vi "TEST - Get Array Element TD.vi"(8 "error in (no error)":errorcluster) -> (0 "error out":errorcluster, 2 "pass":bool)   [LabVIEW 2020, in "test_openg_variant.lvlib"]
uses:
  test_openg_variant.lvlib
  source/library/Type Descriptor.ctl
  <vilib>/addons/_JKI Toolkits/Caraya/classes/Assert/Assert True.vi
  source/library/openg_variant.lvlib
  <vilib>/addons/_JKI Toolkits/Caraya/classes/Test/Test.lvclass
  <vilib>/addons/_JKI Toolkits/Caraya/classes/Assert/Assert.lvclass
panel:
  out "Failures":T2(array[cluster])
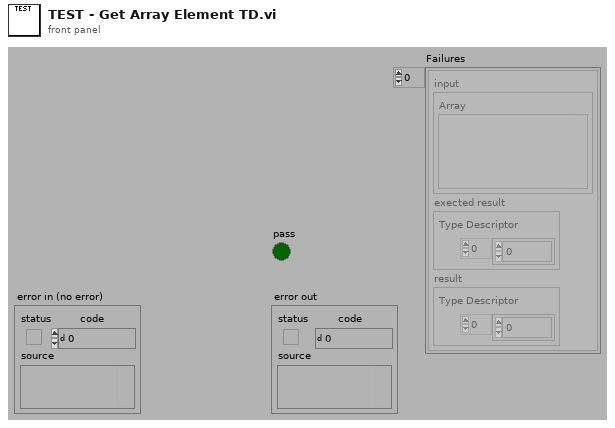
[diagram p1: front panel]
types:
  T1 = typedef "openg_variant.lvlib/Type Descriptor.ctl" = i16[]
  T2 = cluster{"input":cluster{"Array":variant}, "exected result":cluster{"Type Descriptor":T1}, "result":cluster{"Type Descriptor":T1}}[]
  T3 = cluster{"input":cluster{"Array":variant}, "exected result":cluster{"Type Descriptor":T1}, "result":cluster{"Type Descriptor":T1}}
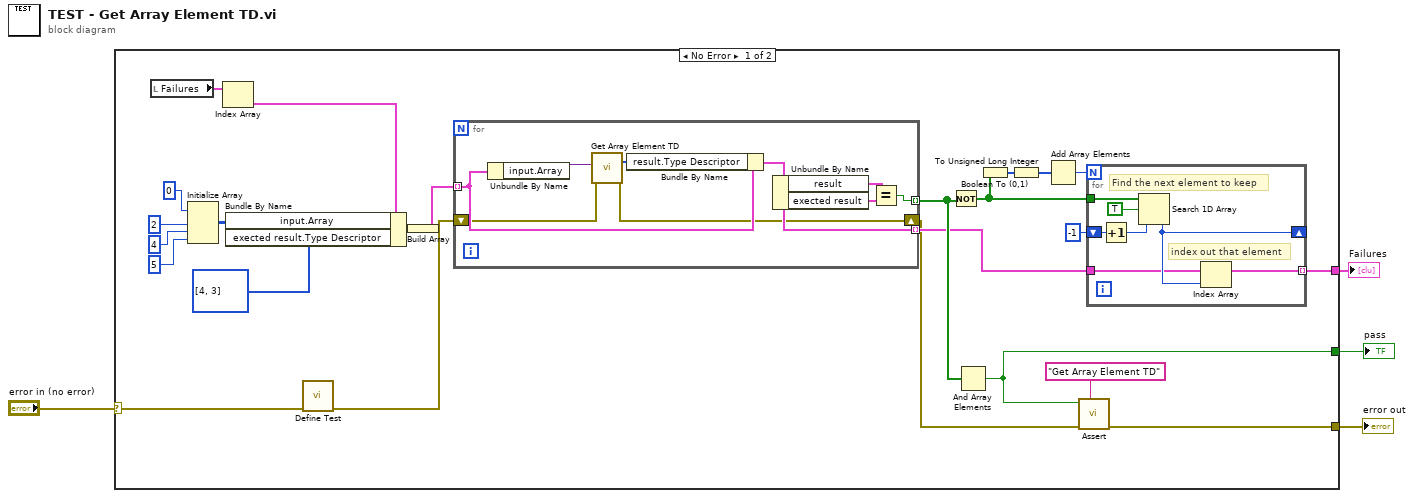
[diagram p0: block diagram]
diagram:
  n1 = case shown="No Error" "error in (no error)" {
    selector: "error in (no error)" -> [w9 w45]
    tunnel: [w5 _] -> w4
    tunnel: [w6 w45] -> w2
    tunnel: [w21 _] -> w1
    frame No Error {
      n2 = local read "Failures"() -> (w18:T2)
      n3 = Initialize Array(0, u32 2 ("Numeric"), 4 ("Numeric"), 5 ("Numeric")) -> (w14:i32[][][])
      n4 = Index Array(array=w18) -> (element=w13:T3)  [unwired: 1 in]
      n5 = Bundle By Name(cluster=w13, "input.Array"=w14, "exected result.Type Descriptor"=T1 [4, 3] ("Type Descriptor")) -> (w20:T3)
      n6 = call <vilib>:"Define Test.vi"("error in (no error)"=w9) -> ("error out"=w8:errorcluster)  [unwired: 9 in, 1 out]
      n7 = Build Array(w20) -> (w19:T2)
      n8 = for {
        tunnel: w19 -> [w43] mode=indexing
        tunnel: [w44] -> w23 mode=indexing
        tunnel: [w42] -> w22 mode=indexing
        shift-right: [w36] -> w7
        shift-left: w8 -> [w37]
        n9 = Unbundle By Name(w43) -> ("input.Array"=w39:variant)
        n10 = call "Get Array Element TD.vi"("error in (no error)"=w37, "Array"=w39) -> ("error out"=w36:errorcluster, "Type Descriptor"=w38:T1)  [unwired: 8 in]
        n11 = Bundle By Name(cluster=w43, "result.Type Descriptor"=w38) -> (w42:T3)
        n12 = Unbundle By Name(w42) -> ("result"=w41:cluster{"Type Descriptor":T1}, "exected result"=w40:cluster{"Type Descriptor":T1})
        n13 = Equal?(x=w41, y=w40) -> (x = y?=w44:bool)
      }
      n14 = Not(x=w23) -> (.not. x?=w25:bool[])
      n15 = And Array Elements(Boolean array=w23) -> (logical AND=w5:bool)
      n16 = Boolean To (0,1)(Boolean=w25) -> (0, 1=w26:i16[])
      n17 = To Unsigned Long Integer(number=w26) -> (unsigned 32bit integer=w24:u32[])
      n18 = Add Array Elements(numeric array=w24) -> (sum=w27:u32)
      n19 = call-poly <vilib>:"Assert.vi"("Label"="Get Array Element TD" ("Label (VI Title)"), "error in (no error)"=w7, "True?"=w5) -> ("error out"=w6:errorcluster)  [unwired: 7 in, 1 out]
      n20 = for {
        N: w27 -> [_]
        tunnel: w22 -> [w31]
        tunnel: w25 -> [w35]
        shift-right: [w32] -> _
        shift-left: -1 ("start index (0)") -> [w33]
        tunnel: [w30] -> w21 mode=indexing
        # "index out that element"
        # "Find the next element to keep"
        n21 = Increment(x=w33) -> (x+1=w29:i32)
        n22 = Search 1D Array(1D array=w35, element=TRUE, start index (0)=w29) -> (index of element=w32:i32)
        n23 = Index Array(array=w31, index=w32) -> (element=w30:T3)
      }
    }
    frame Error {
    }
  }
  "pass" <- w4
  "error out" <- w2
  "Failures" <- w1
